vi "Write Move to Move List.vi"(8 "error in (no error)":errorcluster, 10 "Move":string, 11 "Burrow in":refnum<class "Burrow.lvclass">) -> (0 "error out":errorcluster, 3 "Burrow out":refnum<class "Burrow.lvclass">)   [LabVIEW 2019, in "23.lvlib" / "Burrow.lvclass"]
uses:
  Burrow.lvclass
  Burrow.lvclass/Burrow.ctl
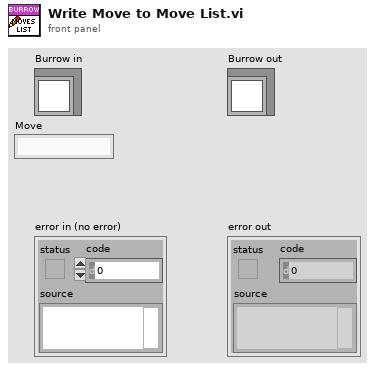
[diagram p1: front panel]
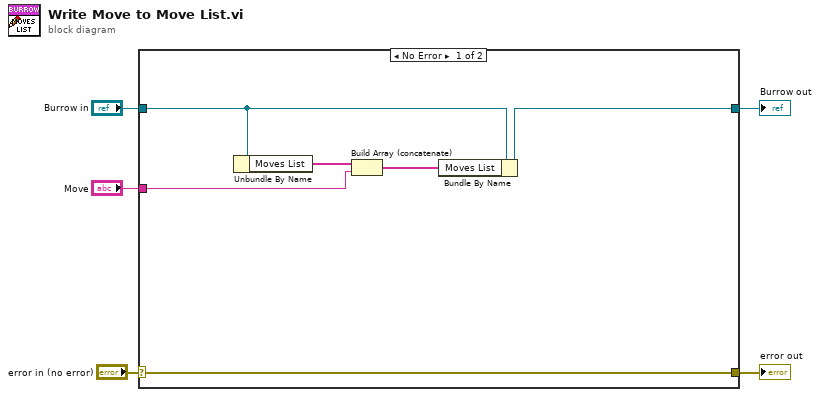
[diagram p0: block diagram]
diagram:
  n1 = case shown="No Error" "error in (no error)" {
    selector: "error in (no error)" -> [w8 w13]
    tunnel: [w8 w13] -> w4
    tunnel: [w7 w12] -> w2
    tunnel: "Burrow in" -> [w11 w12]
    tunnel: "Move" -> [w9 _]
    frame No Error {
      n2 = Unbundle By Name(w11) -> ("Moves List"=w10:string[])
      n3 = Build Array (concatenate)(w10, w9) -> (w6:string[])
      n4 = Bundle By Name(cluster=w11, "Moves List"=w6) -> (w7:refnum<class "Burrow.lvclass">)
    }
    frame Error {
    }
  }
  "error out" <- w4
  "Burrow out" <- w2
